vi "robot_comSUBVI.vi"(8 "error in (no error)":errorcluster, 10 "message":string, 11 "ConnectionID In":refnum<k5>) -> (0 "error IO":errorcluster, 2 "robotmessage":string, 3 "connection ID":refnum<k5>)   [LabVIEW 2022 SP3]
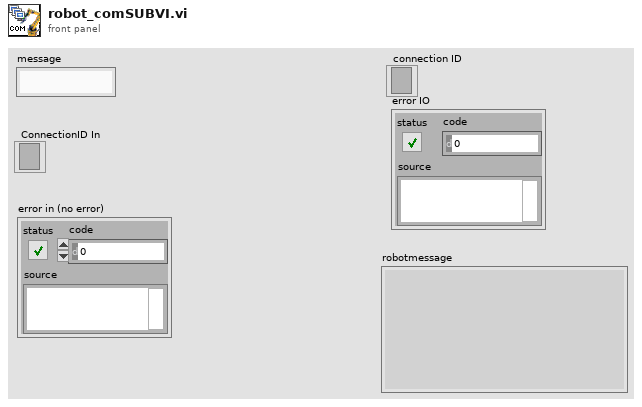
[diagram p1: front panel]
types:
  T1 = enum16{"Standard", "Buffered", "CRLF", "Immediate"}
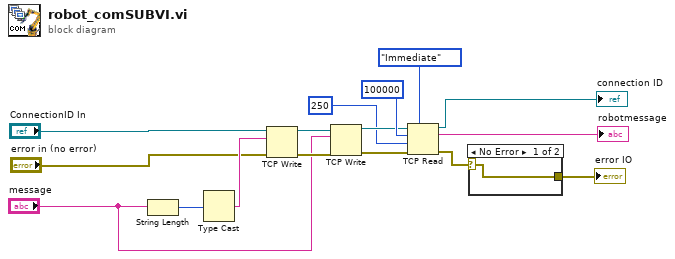
[diagram p0: block diagram]
diagram:
  n1 = String Length(string="message") -> (length=w12:i32)
  n2 = Type Cast(x=w12) -> (*(type *) &x=w11:string)  [unwired: 1 in]
  n3 = TCP Write(connection ID="ConnectionID In", data in=w11, error in (no error)="error in (no error)") -> (connection ID out=w10:refnum<k5>, error out=w9:errorcluster)  [unwired: 1 in, 1 out]
  n4 = TCP Write(connection ID=w10, data in="message", error in (no error)=w9) -> (connection ID out=w7:refnum<k5>, error out=w8:errorcluster)  [unwired: 1 in, 1 out]
  n5 = TCP Read(connection ID=w7, bytes to read=100000, error in (no error)=w8, 7:T1."Immediate" ("mode (standard)"), 9:250 ("timeout ms (25000)")) -> (connection ID out=→"connection ID":refnum<k5>, data out=→"robotmessage":string, error out=w14:errorcluster)
  n6 = case shown="No Error" w14 {
    selector: w14 -> [w17 _]
    tunnel: [w17 _] -> w4
    frame No Error {
    }
    frame Error {
    }
  }
  "error IO" <- w4
